vi "fit magnet to position backup.vi"(8 "error in (no error)":errorcluster, 9 "crossing-2":dbl=-inf, 10 "current crossing":dbl=inf, 11 "display queues":T1) -> (0 "error out":errorcluster, 1 "mean time":dbl format="%0.2f", 2 "z mag and fit":cluster{dbl[], "best nonlinear fit":dbl[]}[](array[cluster]), 3 "mag xy position":cluster{dbl[], dbl[]})   [LabVIEW 2017]
uses:
  typedefs/queue cluster.ctl
  typedefs/reading1.ctl
  typedefs/reading3.ctl
  <vilib>/Analysis/baseanly.llb/Mean (DBL).vi
  <vilib>/gmath/NumericalOptimization/Nonlinear Curve Fit LM formula string.vi
  <vilib>/gmath/NI_Gmath.lvlib
  <vilib>/Analysis/NI_AALBase.lvlib
panel:
  out "XY Graph 2":cluster{dbl[], dbl[]}[](graph)
  out "XY Graph":cluster{dbl[], dbl[]}[](graph)
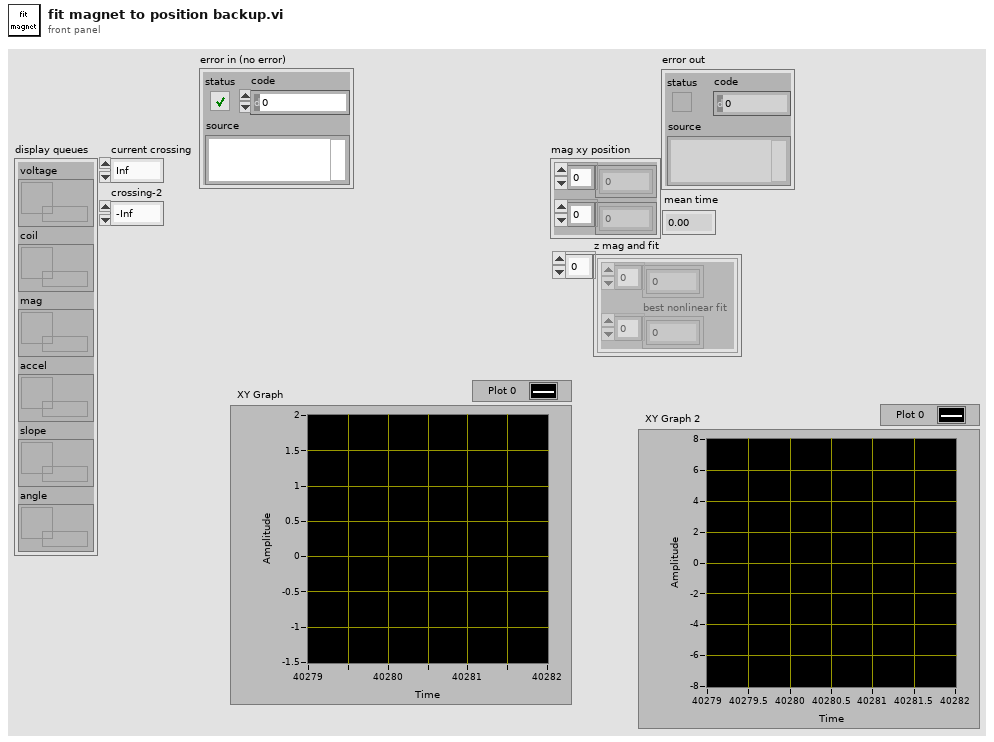
[diagram p1: front panel]
types:
  T1 = typedef "queue cluster.ctl" = cluster{"voltage":refnum<queue>, "coil":refnum<queue>, "mag":refnum<queue>, "accel":refnum<queue>, "slope":refnum<queue>, "angle":refnum<queue>}
  T2 = cluster{"model":string, "Parameters":string[], "x":string}
  T3 = typedef "reading3.ctl" = cluster{"time":dbl, "x":dbl, "y":dbl, "z":dbl, "ms timer":u32}
  T4 = cluster{"time":dbl, "x":dbl, "y":dbl, "z":dbl, "ms timer":dbl}
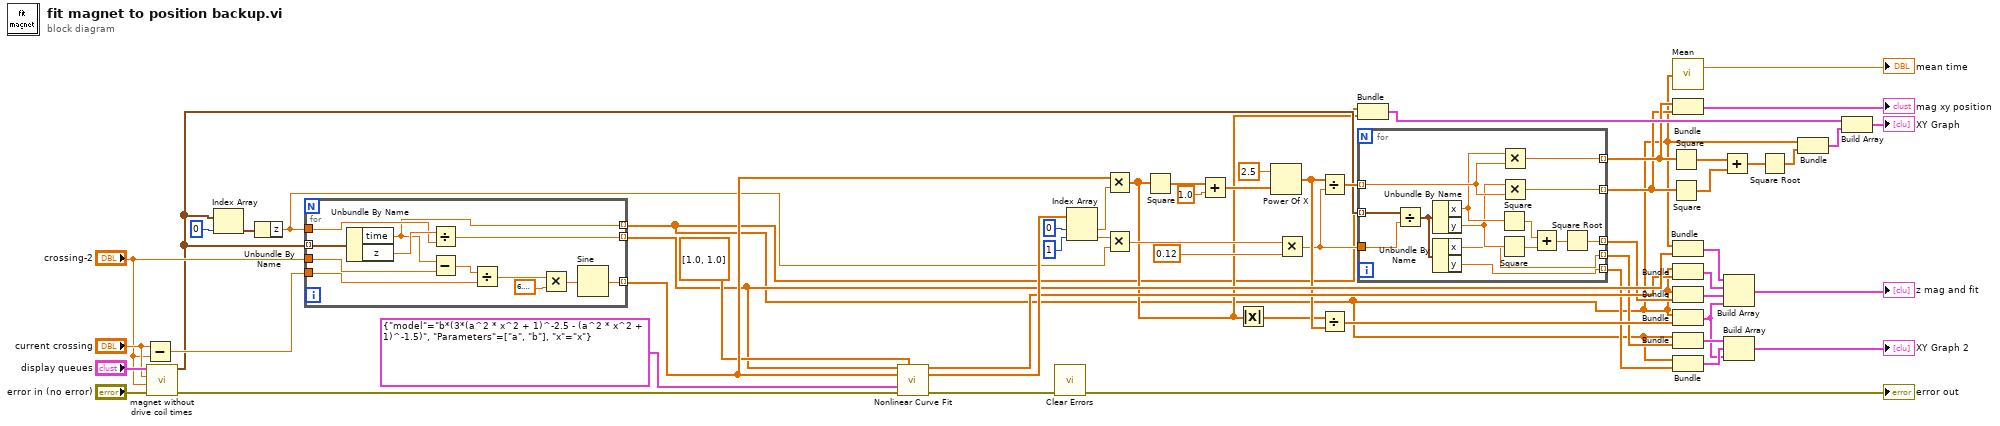
[diagram p0: block diagram]
diagram:
  n1 = Subtract(x="current crossing", y="crossing-2") -> (x-y=w55:dbl)
  n2 = call "magnet without drive coil times.vi"("error in (no error)"="error in (no error)", "min time"="crossing-2", "max time"="current crossing", "display queues"="display queues") -> ("error out"=w50:errorcluster, "mag no drive"=w37:T3[])  [unwired: 5 in, 1 out]
  n3 = Index Array(array=w37, index=0) -> (element=w53:T3)
  n4 = Unbundle By Name(w53) -> ("z"=w40:dbl)
  n5 = for {
    tunnel: w37 -> [w69] mode=indexing
    tunnel: w55 -> [w66]
    tunnel: "crossing-2" -> [w68]
    tunnel: [w59] -> w47 mode=indexing
    tunnel: w40 -> [w62]
    tunnel: [w61] -> w34 mode=indexing
    tunnel: [w58] -> w4 mode=indexing
    n6 = Unbundle By Name(w69) -> ("time"=w58:dbl, "z"=w63:dbl)
    n7 = Divide(x=w63, y=w62) -> (x/y=w61:dbl)
    n8 = Subtract(x=w58, y=w68) -> (x-y=w67:dbl)
    n9 = Divide(x=w67, y=w66) -> (x/y=w65:dbl)
    n10 = Multiply(x=w65, y=6.283185307179586) -> (x*y=w60:dbl)
    n11 = Sine(x=w60) -> (sin(x)=w59:dbl)
  }
  n12 = call-poly <vilib>:"Nonlinear Curve Fit.vi"("Y"=w34, "initial parameters"=dbl[] [1.0, 1.0], "X"=w47, "model description"=T2 {"model"="b*(3*(a^2 * x^2 + 1)^-2.5 - (a^2 * x^2 + 1)^-1.5)", "Parameters"=["a", "b"], "x"="x"}, "error in (no error)"=w50) -> ("best nonlinear fit"=w33:dbl[], "best fit parameters"=w49:dbl[], "error out"=w28:errorcluster)  [unwired: 6 in, 2 out]
  n13 = call <vilib>:"Clear Errors.vi"("error in (no error)"=w28) -> ("error out"=→"error out":errorcluster)  [unwired: 5 in, 1 out]
  n14 = Index Array(array=w49, index #1=0 ("index"), index #2=1 ("index")) -> (element #1=w48:dbl, element #2=w41:dbl)
  n15 = Multiply(x=w47, y=w48) -> (x*y=w20:dbl[])
  n16 = Multiply(x=w41, y=w40) -> (x*y=w27:dbl)
  n17 = Square(x=w20) -> (x^2=w25:dbl[])
  n18 = Add(x=w25, y=1.0) -> (x+y=w45:dbl[])
  n19 = Absolute Value(x=w20) -> (abs(x)=w21:dbl[])
  n20 = Power Of X(1:w45, 2:2.5) -> (0:w26:dbl[])
  n21 = Multiply(x=w27, y=0.12) -> (x*y=w12:dbl)
  n22 = Divide(x=w26, y=w12) -> (x/y=w38:dbl[])
  n23 = Divide(x=w21, y=w26) -> (x/y=w23:dbl[])
  n24 = Bundle(w4, w20) -> (w19:cluster{dbl[], dbl[]})  [unwired: 1 in]
  n25 = for {
    tunnel: w38 -> [w76] mode=indexing
    tunnel: w37 -> [w73] mode=indexing
    tunnel: [w83] -> w6 mode=indexing
    tunnel: [w82] -> w5 mode=indexing
    tunnel: w12 -> [w80]
    tunnel: [w77] -> w24 mode=indexing
    tunnel: [w71] -> w18 mode=indexing
    tunnel: [w72] -> w17 mode=indexing
    n26 = Divide(x=w73, y=w80) -> (x/y=w70:T4)
    n27 = Unbundle By Name(w70) -> ("x"=w75:dbl, "y"=w74:dbl)
    n28 = Unbundle By Name(w70) -> ("x"=w71:dbl, "y"=w72:dbl)
    n29 = Square(x=w75) -> (x^2=w81:dbl)
    n30 = Square(x=w74) -> (x^2=w79:dbl)
    n31 = Multiply(x=w75, y=w76) -> (x*y=w83:dbl)
    n32 = Multiply(x=w74, y=w76) -> (x*y=w82:dbl)
    n33 = Add(x=w81, y=w79) -> (x+y=w78:dbl)
    n34 = Square Root(x=w78) -> (sqrt(x)=w77:dbl)
  }
  n35 = Square(x=w6) -> (x^2=w9:dbl[])
  n36 = Square(x=w5) -> (x^2=w8:dbl[])
  n37 = call-poly <vilib>:"Mean.vi"("X"=w4) -> ("mean"=→"mean time":dbl)  [unwired: 1 out]
  n38 = Bundle(w6, w5) -> (→"mag xy position":cluster{dbl[], dbl[]})  [unwired: 1 in]
  n39 = Bundle(w4, w34) -> (w32:cluster{dbl[], dbl[]})  [unwired: 1 in]
  n40 = Bundle(w4, "best nonlinear fit"=w33) -> (w31:cluster{dbl[], "best nonlinear fit":dbl[]})  [unwired: 1 in]
  n41 = Bundle(w4, w24) -> (w22:cluster{dbl[], dbl[]})  [unwired: 1 in]
  n42 = Bundle(w4, w23) -> (w13:cluster{dbl[], dbl[]})  [unwired: 1 in]
  n43 = Bundle(w4, w18) -> (w16:cluster{dbl[], dbl[]})  [unwired: 1 in]
  n44 = Bundle(w4, w17) -> (w15:cluster{dbl[], dbl[]})  [unwired: 1 in]
  n45 = Add(x=w9, y=w8) -> (x+y=w7:dbl[])
  n46 = Build Array(w32, w31, w22, w13) -> (→"z mag and fit":cluster{dbl[], "best nonlinear fit":dbl[]}[])
  n47 = Build Array(w16, w15, w13) -> (→"XY Graph 2":cluster{dbl[], dbl[]}[])
  n48 = Square Root(x=w7) -> (sqrt(x)=w3:dbl[])
  n49 = Bundle(w4, w3) -> (w1:cluster{dbl[], dbl[]})  [unwired: 1 in]
  n50 = Build Array(w19, w1) -> (→"XY Graph":cluster{dbl[], dbl[]}[])
